vi "UDP_string_to_DBL.vi"(1 "input string":string) -> (0 "output number":i32)   [LabVIEW 2012]
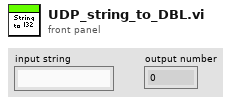
[diagram p1: front panel]
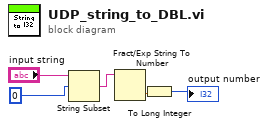
[diagram p0: block diagram]
diagram:
  n1 = String Subset(string="input string", offset (0)=0 ("offset")) -> (substring=w4:string)  [unwired: 1 in]
  n2 = Fract/Exp String To Number(string=w4) -> (number=w2:dbl)  [unwired: 3 in, 1 out]
  n3 = To Long Integer(number=w2) -> (32bit integer=→"output number":i32)
